vi "PH_ImageOperator.Lev-Mar abx.vi"(4 "Order of GAUSSian function":i32, 5 "No Offset?":bool, 6 "Standard Deviation":dbl[](array[numeric]) format="%0.2f", 7 "Coefficients":dbl[](array[numeric]) format="%0.2f", 8 "Y":dbl[](array[numeric]) format="%0.2f", 9 "X":dbl[](array[numeric]) format="%0.2f") -> (0 "chiSqr":dbl format="%0.2f", 1 "Beta":dbl[](array[numeric]) format="%0.2f", 3 "Alpha":dbl[][](array[numeric]) format="%0.2f")   [LabVIEW 2014, in "PH_ImageOperator.lvlib"]
uses:
  PH_ImageOperator.lvlib
panel:
  # "Lev-Mar\nabx"
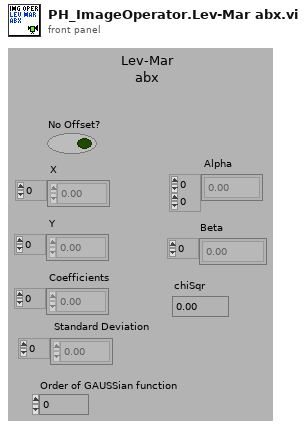
[diagram p1: front panel]
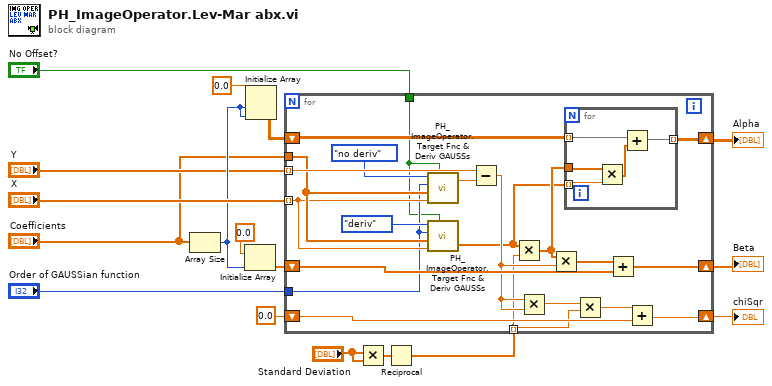
[diagram p0: block diagram]
diagram:
  n1 = Array Size(array="Coefficients") -> (size(s)=w15:i32)
  n2 = Initialize Array(0.0, w15) -> (w14:dbl[])
  n3 = Initialize Array(0.0, w15, w15) -> (w13:dbl[][])
  n4 = Multiply(x="Standard Deviation", y="Standard Deviation") -> (x*y=w5:dbl[])
  n5 = Reciprocal(x=w5) -> (1/x=w3:dbl[])
  n6 = for {
    tunnel: "X" -> [w26] mode=indexing
    shift-right: [w33] -> w11
    shift-left: w14 -> [w35]
    shift-right: [w30] -> w8
    shift-left: w13 -> [w31]
    shift-right: [w29] -> w4
    shift-left: 0.0 -> [w37]
    tunnel: "Y" -> [w36] mode=indexing
    tunnel: "Coefficients" -> [w27]
    tunnel: w3 -> [w23] mode=indexing
    tunnel: "Order of GAUSSian function" -> [w19]
    tunnel: "No Offset?" -> [w18]
    n7 = call "PH_ImageOperator.Target Fnc & Deriv GAUSSs.vi"("Flag"=enum16{"no deriv", "deriv"}."no deriv", "Order of GAUSSian function"=w19, "Coefficients"=w27, "X"=w26, "No Offset?"=w18) -> ("Y"=w28:dbl)  [unwired: 1 out]
    n8 = call "PH_ImageOperator.Target Fnc & Deriv GAUSSs.vi"("Flag"=enum16{"no deriv", "deriv"}."deriv", "Order of GAUSSian function"=w19, "Coefficients"=w27, "X"=w26, "No Offset?"=w18) -> ("Derivatives"=w22:dbl[])  [unwired: 1 out]
    n9 = Subtract(x=w36, y=w28) -> (x-y=w32:dbl)
    n10 = Multiply(x=w22, y=w23) -> (x*y=w25:dbl[])
    n11 = Multiply(x=w32, y=w32) -> (x*y=w38:dbl)
    n12 = Multiply(x=w25, y=w32) -> (x*y=w34:dbl[])
    n13 = for {
      tunnel: w25 -> [w43]
      tunnel: w31 -> [w42] mode=indexing
      tunnel: [w40] -> w30 mode=indexing
      tunnel: w22 -> [w39] mode=indexing
      n14 = Multiply(x=w43, y=w39) -> (x*y=w41:dbl[])
      n15 = Add(x=w42, y=w41) -> (x+y=w40:dbl[])
    }
    n16 = Multiply(x=w38, y=w23) -> (x*y=w24:dbl)
    n17 = Add(x=w34, y=w35) -> (x+y=w33:dbl[])
    n18 = Add(x=w24, y=w37) -> (x+y=w29:dbl)
  }
  "Alpha" <- w8
  "Beta" <- w11
  "chiSqr" <- w4
